vi "Initial State Example.vi"() -> ()   [LabVIEW 2013]
uses:
  Initial State LabVIEW SDK/Custom Data Types/IS Data Point TypeDef (String).ctl
  Initial State LabVIEW SDK/IS PolyVI Instance DBL To JSON Cluster .vi
  Initial State LabVIEW SDK/Data Helpers/IS PolyVI Instance Bool To JSON Cluster .vi
  Initial State LabVIEW SDK/Data Helpers/IS PolyVI Instance String to JSON Cluster.vi
panel:
  out "Buffer Size":i32
  in  "stop":bool
  out "Waveform Chart":dbl(graph)=0.6082396240250167
  in  "Bucket Name (Optional)":string="LabVIEW Example Bucket"
  in  "Access Key":string="FakeFakeVj0GLMeSHRkyOEAPFGhzWEmw"
  out "Response Headers":string
  out "Response Body":string
  # "Initial State Streaming LabVIEW Example"
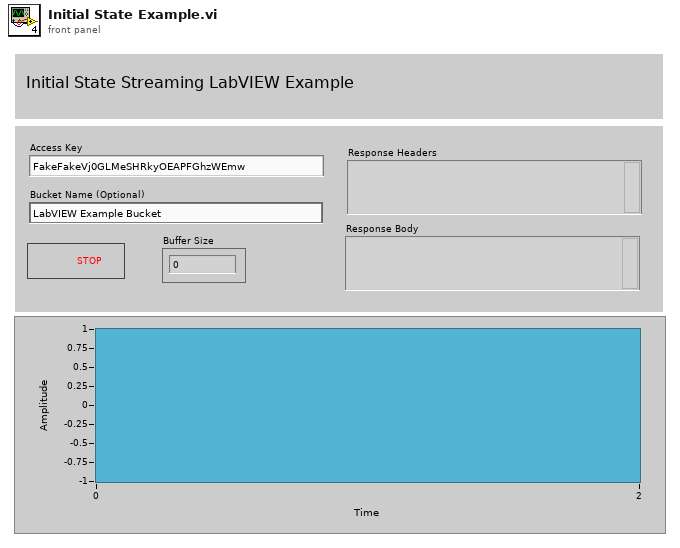
[diagram p1: front panel]
types:
  T1 = typedef "IS Data Point TypeDef (String).ctl" = cluster{"key":string, "value":string, "epoch":dbl}
  T2 = typedef "IS Session.ctl" = cluster{"Access Key":string, "HTTP Client Handle":T3}
  T3 = typedef "LabVIEWHTTPClient.lvlib/ClientHandle.ctl" = refnum<k1>
  T4 = typedef "IS Bucket Session.ctl" = cluster{"Bucket Key":string}
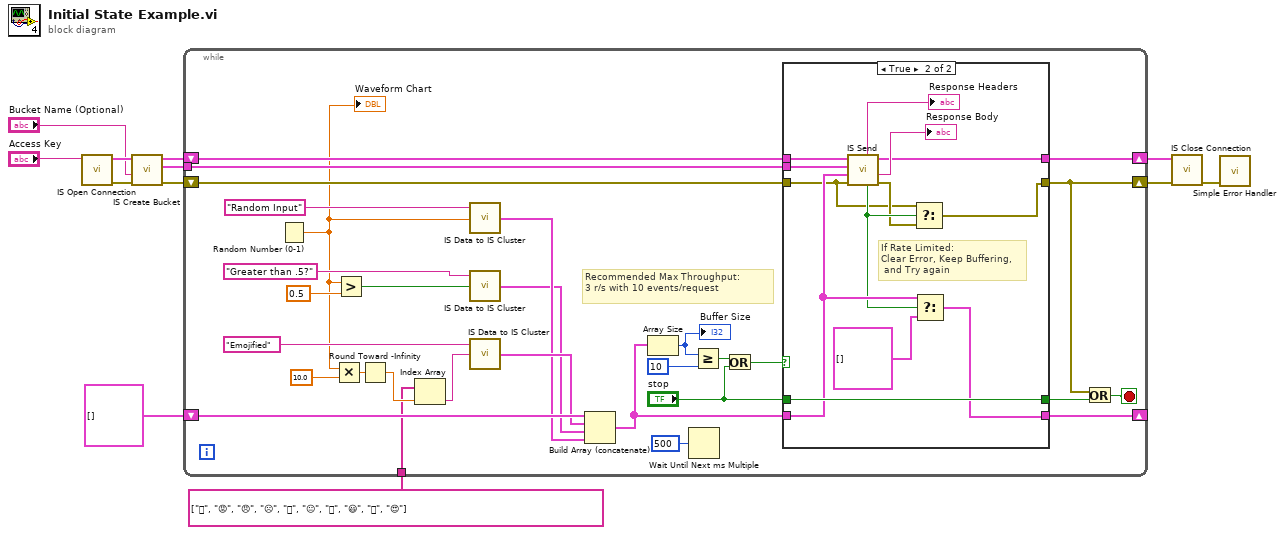
[diagram p0: block diagram]
diagram:
  n1 = call "IS Open Connection.vi"("Access Key"="Access Key") -> ("error out"=w10:errorcluster, "IS Session"=w12:T2)  [unwired: 9 in]
  n2 = call "IS Create Bucket.vi"("error in (no error)"=w10, "Bucket Name (Optional)"="Bucket Name (Optional)", "IS Session In"=w12) -> ("error IO"=w4:errorcluster, "IS Bucket Session"=w7:T4, "IS Session Out"=w6:T2)  [unwired: 6 in]
  n3 = while {
    tunnel: w7 -> [w39]
    shift-right: [w42] -> w2
    shift-left: w6 -> [w41]
    shift-right: [w22] -> w1
    shift-left: w4 -> [w40]
    shift-right: [w37] -> _
    shift-left: T1[] [] -> [w38]
    tunnel: string[] ["🤬", "😡", "😠", "☹️", "🙁", "😐", "🙂", "😃", "🤩", "😍"] -> [w27]
    stop <- w21 stop-if-true
    # "Recommended Max Throughput: \n3 r/s with 10 events/request"
    n4 = Random Number (0-1)() -> (number: 0 to 1=w16:dbl)
    "Waveform Chart" <- w16
    n5 = Multiply(x=w16, y=10.0) -> (x*y=w30:dbl)
    n6 = Greater?(x=w16, y=0.5) -> (0:w15:bool)
    n7 = Round Toward -Infinity(1:w30) -> (0:w28:dbl)
    n8 = Index Array(array=w27, index=w28) -> (element=w14:string)
    n9 = call-poly "IS Data to IS Cluster.vi"("Stream Value"=w16, "Stream Key"="Random Input") -> ("JSON Cluster Array out"=w24:T1[])  [unwired: 3 in]
    n10 = call-poly "IS Data to IS Cluster.vi"("Stream Value"=w15, "Stream Key"="Greater than .5?") -> ("JSON Cluster Array out"=w23:T1[])  [unwired: 3 in]
    n11 = call-poly "IS Data to IS Cluster.vi"("Stream Value"=w14, "Stream Key"="Emojified") -> ("JSON Cluster Array out"=w25:T1[])  [unwired: 3 in]
    n12 = Build Array (concatenate)(w38, w25, w23, w24) -> (w36:T1[])
    n13 = Array Size(array=w36) -> (size(s)=w35:i32)
    "Buffer Size" <- w35
    n14 = Wait Until Next ms Multiple(millisecond multiple=u32 500) -> ()  [unwired: 1 out]
    n15 = Greater Or Equal?(x=w35, y=10) -> (x >= y?=w19:bool)
    n16 = Or(x=w19, y="stop") -> (x .or. y?=w18:bool)
    n17 = case shown="True" w18 {
      tunnel: [w46 w55] -> w42
      tunnel: [w45 w47] -> w22
      tunnel: w41 -> [w46 w59]
      tunnel: w40 -> [w45 w48]
      tunnel: w39 -> [_ w58]
      tunnel: w36 -> [w44 w52]
      tunnel: [w44 w51] -> w37
      tunnel: "stop" -> [w43 w56]
      tunnel: [w43 w56] -> w20
      frame False {
      }
      frame True {
        # "If Rate Limited: \nClear Error, Keep Buffering,\n and Try again"
        n18 = call "IS Send.vi"("error in (no error)"=w48, "JSON Custer Array in"=w52, "IS Bucket Session"=w58, "IS Session in"=w59) -> ("Error out"=w49:errorcluster, "Response Body"=→"Response Body":string, "IS Session out"=w55:T2, "Rate Limit Reached?"=w50:bool, "Response Headers"=→"Response Headers":string)  [unwired: 2 in, 1 out]
        n19 = Select(t=w48, s=w50, f=w49) -> (s? t:f=w47:errorcluster)
        n20 = Select(t=w52, s=w50, f=T1[] []) -> (s? t:f=w51:T1[])
      }
    }
    n21 = Or(x=w22, y=w20) -> (x .or. y?=w21:bool)
  }
  n22 = call "IS Close Connection.vi"("error in (no error)"=w1, "IS Session In"=w2) -> ("error out"=w9:errorcluster)  [unwired: 9 in]
  n23 = call <vilib>:"Simple Error Handler.vi"("error in (no error)"=w9) -> ()  [unwired: 4 in, 5 out]
